vi "Rec Move To Previous Record (R).vi"(8 "error in (no error)":errorcluster, 11 "recordset reference":T1) -> (0 "error out":errorcluster, 3 "recordset reference out":T1)   [LabVIEW 2017, in "NI_Database_API.lvlib"]
doc: "Moves the cursor to point to the previous record in the recordset. You cannot use this VI with a forward-only cursor. Wire data to the reference input to determine the polymorphic instance to use or manually select the instance."
uses:
  <vilib>/addons/database/NI_Database_API.lvlib
  <vilib>/addons/database/Recordset.llb/Rec ObjectReference.ctl
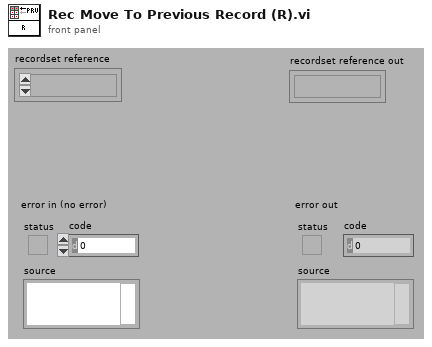
[diagram p1: front panel]
types:
  T1 = typedef "NI_Database_API.lvlib/Rec ObjectReference.ctl" = refnum<k1>
  T2 = typedef "NI_Database_API.lvlib/Rec DataMembers.ctl" = cluster{"ADODB._Recordset":refnum<k7>, "Connection":T3}
  T3 = typedef "NI_Database_API.lvlib/Conn ObjectReference.ctl" = refnum<k1>
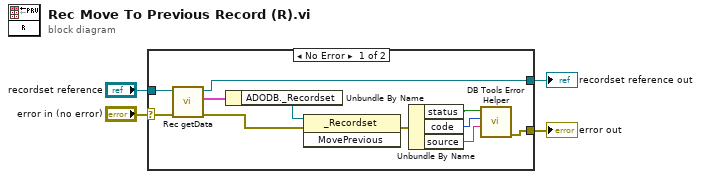
[diagram p0: block diagram]
diagram:
  n1 = case shown="No Error" "error in (no error)" {
    selector: "error in (no error)" -> [w5 w17]
    tunnel: [w14 w16] -> w4
    tunnel: "recordset reference" -> [w13 w16]
    tunnel: [w6 w17] -> w2
    frame No Error {
      n2 = call <vilib>:"Rec getData.vi"("error in (no error)"=w5, "recordset reference"=w13) -> ("error out"=w12:errorcluster, "data"=w15:T2, "recordset reference out"=w14:T1)  [unwired: 3 out]
      n3 = Unbundle By Name(w15) -> ("ADODB._Recordset"=w11:refnum<k7>)
      n4 = invoke class="_Recordset" method="MovePrevious"(reference=w11, error in=w12) -> (error out=w7:errorcluster)  [unwired: 1 in, 2 out]
      n5 = Unbundle By Name(w7) -> ("status"=w9:bool, "code"=w8:i32, "source"=w10:string)
      n6 = call <vilib>:"DB Tools Error Helper.vi"("source"=w10, "code"=w8, "status"=w9) -> ("error out"=w6:errorcluster)  [unwired: 1 in, 7 out]
    }
    frame Error {
    }
  }
  "recordset reference out" <- w4
  "error out" <- w2
